vi "media e deviazione.vi"(0 "2D array":dbl[][](array[numeric])) -> (6 "Mean Array - Active Power":dbl[](array[numeric]), 7 "Dev Array - Active Power":dbl[](array[numeric]))   [LabVIEW 2018]
uses:
  <vilib>/Analysis/NI_AALBase.lvlib
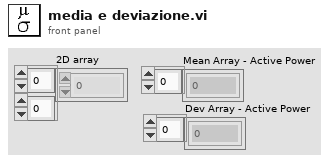
[diagram p1: front panel]
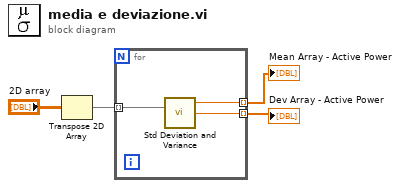
[diagram p0: block diagram]
diagram:
  n1 = Transpose 2D Array(2D array="2D array") -> (transposed array=w3:dbl[][])
  n2 = for {
    tunnel: w3 -> [w7] mode=indexing
    tunnel: [w6] -> w2 mode=indexing
    tunnel: [w5] -> w1 mode=indexing
    n3 = call <vilib>:"Std Deviation and Variance.vi"("X"=w7) -> ("mean"=w6:dbl, "standard deviation"=w5:dbl)  [unwired: 1 in, 1 out]
  }
  "Mean Array - Active Power" <- w2
  "Dev Array - Active Power" <- w1
